vi "6-9.vi"() -> ()   [LabVIEW 2017]
panel:
  out "data":string
  in  "file path (use dialog)":path
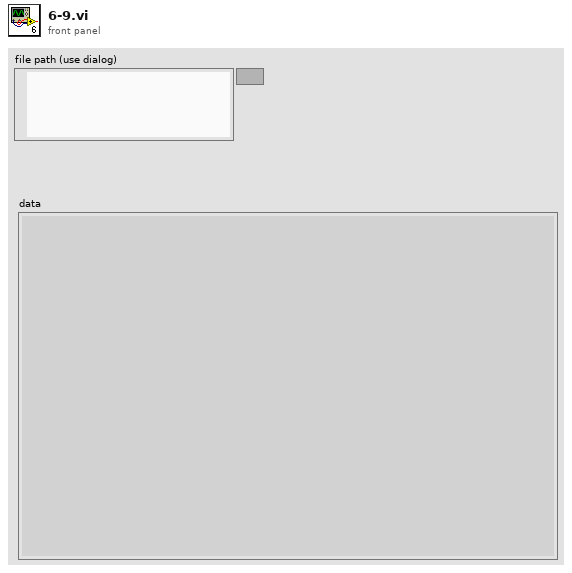
[diagram p1: front panel]
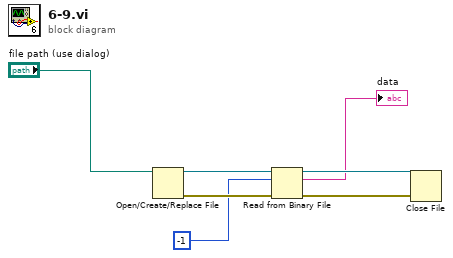
[diagram p0: block diagram]
diagram:
  n1 = Open/Create/Replace File(file path (use dialog)="file path (use dialog)") -> (refnum out=w5:refnum<file>, error out=w6:errorcluster)  [unwired: 5 in, 1 out]
  n2 = Read from Binary File(8:w6, 10:-1 ("count (1)"), 11:w5) -> (0:w4:errorcluster, 2:→"data":string, 3:w3:refnum<file>)  [unwired: 3 in, 1 out]
  n3 = Close File(refnum=w3, error in=w4) -> ()  [unwired: 2 out]
